vi "Wait for MEssages.vi"(8 "error in (no error)":errorcluster, 11 "object in":refnum<class "JuPyter_Client.lvclass">) -> (0 "error out":errorcluster, 2 "Event Registration Refnum":refnum<event-registration>, 3 "object out":refnum<class "JuPyter_Client.lvclass">)   [LabVIEW 2018, in "JuPyter_Client.lvclass"]
doc: "Polls the IOPub socket and waits for incoming messages and then passes them to the event queue"
uses:
  JuPyter_Client.lvclass
  Base Classes/Message Class/Message Class.lvclass
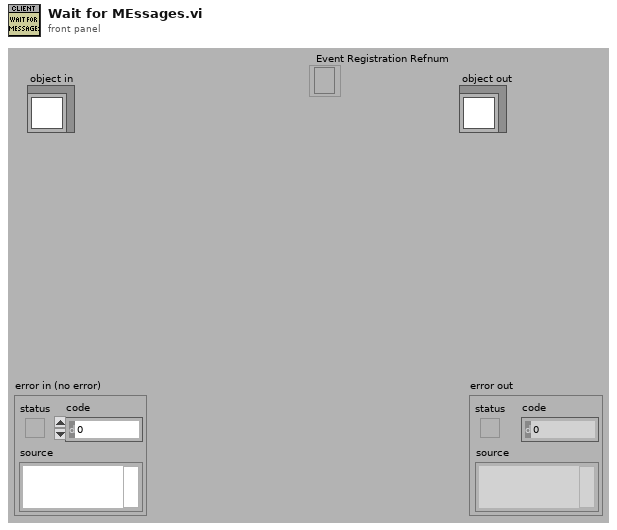
[diagram p1: front panel]
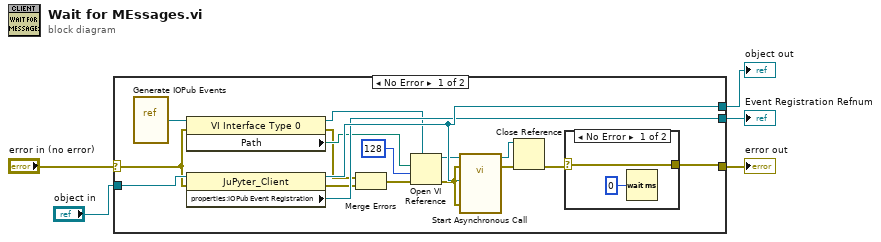
[diagram p0: block diagram]
diagram:
  n1 = case shown="No Error" "error in (no error)" {
    selector: "error in (no error)" -> [w12 w27]
    tunnel: [w6 w27] -> w4
    tunnel: [w20 w26] -> w2
    tunnel: "object in" -> [w22 w26]
    tunnel: [w19 _] -> w1
    frame No Error {
      n2 = vi-ref "Generate IOPub Events.vi"() -> (w21:refnum<vi>)
      n3 = property class="VI Interface Type 0"(reference=w21, error in=w12) -> (reference out=w14:refnum<vi>, error out=w10:errorcluster, "Path"=w13:path)
      n4 = property class="JuPyter_Client"(reference=w22, error in=w12) -> (reference out=w20:refnum<class "JuPyter_Client.lvclass">, error out=w16:errorcluster, "properties:IOPub Event Registration"=w19:refnum<event-registration>)
      n5 = Merge Errors(w10, w16) -> (w11:errorcluster)
      n6 = Open VI Reference(type specifier VI Refnum (for type only)=w14, vi path=w13, options=128, error in (no error)=w11) -> (vi reference=w18:refnum<vi>, error out=w15:errorcluster)  [unwired: 2 in]
      n7 = call-by-ref "Start Asynchronous Call"(reference=w18, error in=w15, 8:"error in (no error)"=w15, "object in"=w20) -> (reference out=w9:refnum<vi>, error out=w8:errorcluster)  [unwired: 8 in, 2 out]
      n8 = Close Reference(reference=w9, error in (no error)=w8) -> (error out=w7:errorcluster)
      n9 = case shown="No Error" w7 {
        selector: w7 -> [w24 w25]
        tunnel: [w24 w25] -> w6
        frame No Error {
          n10 = Wait (ms)(milliseconds to wait=u32 0) -> ()  [unwired: 1 out]
        }
        frame Error {
        }
      }
    }
    frame Error {
    }
  }
  "error out" <- w4
  "object out" <- w2
  "Event Registration Refnum" <- w1
